vi "input.vi"(2 "r":bool, 3 "-":bool, 4 "keys":T2) -> (0 "minus":bool, 1 "output":T1)   [LabVIEW 2013]
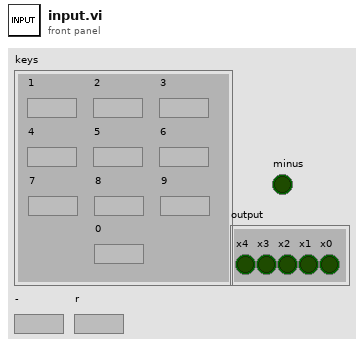
[diagram p1: front panel]
types:
  T1 = cluster{"x4":bool, "x3":bool, "x2":bool, "x1":bool, "x0":bool}
  T2 = cluster{"1":bool, "2":bool, "3":bool, "4":bool, "5":bool, "6":bool, "7":bool, "8":bool, "9":bool, "0":bool}
  T3 = cluster{"x3":bool, "x2":bool, "x1":bool, "x0":bool}
  T4 = cluster{"Y3":bool, "Y2":bool, "Y1":bool, "Y0":bool}
  T5 = cluster{"R4":bool, "R3":bool, "R2":bool, bool, "R0":bool}
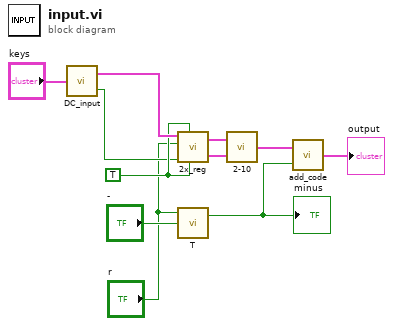
[diagram p0: block diagram]
diagram:
  w10 = TRUE
  n1 = call "DC_input.vi"("input"="keys") -> ("output"=w11:T3, "tick"=w5:bool)
  n2 = call "2x_reg.vi"("WR"=w10, "RD"=w10, "C"=w5, "R"="r", "I"=w11) -> ("O_2"=w9:T4, "O_1"=w8:T4)  [unwired: 1 in]
  n3 = call "T.vi"("T"="-", "R"="r") -> ("Q"=w3:bool)  [unwired: 1 in, 1 out]
  "minus" <- w3
  n4 = call "2-10.vi"("input_decimals"=w9, "input_minors"=w8) -> ("output"=w4:T1)
  n5 = call "add_code.vi"("add_code"=w3, "A"=w4) -> ("Result"=→"output":T5)
